vi "FTW-Linker-DecodeBitmap.vi"(7 "LinkerInfo":T7 {"iState" format="%08x"; "iStyle" format="%08x"; "wStyle" format="%08x"; "buttons" format="%08x"; "viflags" format="%08x"; "viflags2" format="%08x"}) -> (3 "iState":T6, 4 "viflags":T5, 6 "viflags2":T4, 8 "All Flags":bool[](array[boolean]), 10 "iStyle":T3, 14 "buttons":T1, 15 "wStyle":T2)   [LabVIEW 2015]
uses:
  FTW-Linker-LinkerInfoStructure.ctl
  FTW-Linker-LabVIEWFiletype.ctl
  FTW-Linker-Flags-iState.ctl
  FTW-Linker-Flags-viflags.ctl
  FTW-Linker-Flags-viflags2.ctl
  FTW-Linker-Flags-iStyle.ctl
  FTW-Linker-Flags-wStyle.ctl
  FTW-Linker-Flags-buttons.ctl
panel:
  # "Inputs"
  # "Outputs"
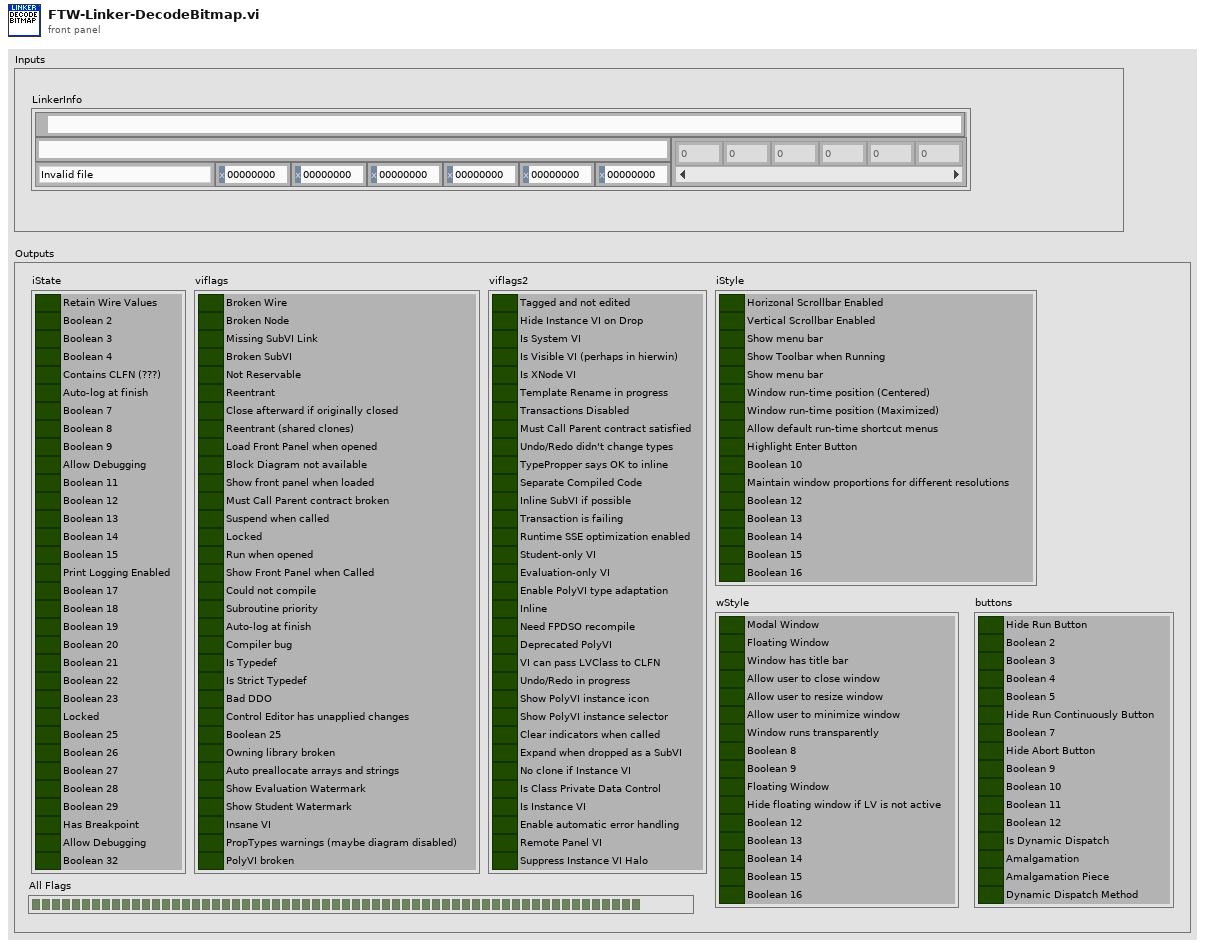
[diagram p1: front panel]
types:
  T1 = typedef "FTW-Linker-Flags-buttons.ctl" = cluster{"Hide Run Button":bool, "Boolean 2":bool, "Boolean 3":bool, "Boolean 4":bool, "Boolean 5":bool, "Hide Run Continuously Button":bool, "Boolean 7":bool, "Hide Abort Button":bool, "Boolean 9":bool, "Boolean 10":bool, "Boolean 11":bool, "Boolean 12":bool, "Is Dynamic Dispatch":bool, "Amalgamation":bool, "Amalgamation Piece":bool, "Dynamic Dispatch Method":bool}
  T2 = typedef "FTW-Linker-Flags-wStyle.ctl" = cluster{"Modal Window":bool, "Floating Window":bool, "Window has title bar":bool, "Allow user to close window":bool, "Allow user to resize window":bool, "Allow user to minimize window":bool, "Window runs transparently":bool, "Boolean 8":bool, "Boolean 9":bool, "Floating Window":bool, "Hide floating window if LV is not active":bool, "Boolean 12":bool, "Boolean 13":bool, "Boolean 14":bool, "Boolean 15":bool, "Boolean 16":bool}
  T3 = typedef "FTW-Linker-Flags-iStyle.ctl" = cluster{"Horizonal Scrollbar Enabled":bool, "Vertical Scrollbar Enabled":bool, "Show menu bar":bool, "Show Toolbar when Running":bool, "Show menu bar":bool, "Window run-time position (Centered)":bool, "Window run-time position (Maximized)":bool, "Allow default run-time shortcut menus":bool, "Highlight Enter Button":bool, "Boolean 10":bool, "Maintain window proportions for different resolutions":bool, "Boolean 12":bool, "Boolean 13":bool, "Boolean 14":bool, "Boolean 15":bool, "Boolean 16":bool}
  T4 = typedef "FTW-Linker-Flags-viflags2.ctl" = cluster{"Tagged and not edited":bool, "Hide Instance VI on Drop":bool, "Is System VI":bool, "Is Visible VI (perhaps in hierwin)":bool, "Is XNode VI":bool, "Template Rename in progress":bool, "Transactions Disabled":bool, "Must Call Parent contract satisfied":bool, "Undo/Redo didn't change types":bool, "TypePropper says OK to inline":bool, "Separate Compiled Code":bool, "Inline SubVI if possible":bool, "Transaction is failing":bool, "Runtime SSE optimization enabled":bool, "Student-only VI":bool, "Evaluation-only VI":bool, "Enable PolyVI type adaptation":bool, "Inline":bool, "Need FPDSO recompile":bool, "Deprecated PolyVI":bool, "VI can pass LVClass to CLFN":bool, "Undo/Redo in progress":bool, "Show PolyVI instance icon":bool, "Show PolyVI instance selector":bool, "Clear indicators when called":bool, "Expand when dropped as a SubVI":bool, "No clone if Instance VI":bool, "Is Class Private Data Control":bool, "Is Instance VI":bool, "Enable automatic error handling":bool, "Remote Panel VI":bool, "Suppress Instance VI Halo":bool}
  T5 = typedef "FTW-Linker-Flags-viflags.ctl" = cluster{"Broken Wire":bool, "Broken Node":bool, "Missing SubVI Link":bool, "Broken SubVI":bool, "Not Reservable":bool, "Reentrant":bool, "Close afterward if originally closed":bool, "Reentrant (shared clones)":bool, "Load Front Panel when opened":bool, "Block Diagram not available":bool, "Show front panel when loaded":bool, "Must Call Parent contract broken":bool, "Suspend when called":bool, "Locked":bool, "Run when opened":bool, "Show Front Panel when Called":bool, "Could not compile":bool, "Subroutine priority":bool, "Auto-log at finish":bool, "Compiler bug":bool, "Is Typedef":bool, "Is Strict Typedef":bool, "Bad DDO":bool, "Control Editor has unapplied changes":bool, "Boolean 25":bool, "Owning library broken":bool, "Auto preallocate arrays and strings":bool, "Show Evaluation Watermark":bool, "Show Student Watermark":bool, "Insane VI":bool, "PropTypes warnings (maybe diagram disabled)":bool, "PolyVI broken":bool}
  T6 = typedef "FTW-Linker-Flags-iState.ctl" = cluster{"Retain Wire Values":bool, "Boolean 2":bool, "Boolean 3":bool, "Boolean 4":bool, "Contains CLFN (???)":bool, "Auto-log at finish":bool, "Boolean 7":bool, "Boolean 8":bool, "Boolean 9":bool, "Allow Debugging":bool, "Boolean 11":bool, "Boolean 12":bool, "Boolean 13":bool, "Boolean 14":bool, "Boolean 15":bool, "Print Logging Enabled":bool, "Boolean 17":bool, "Boolean 18":bool, "Boolean 19":bool, "Boolean 20":bool, "Boolean 21":bool, "Boolean 22":bool, "Boolean 23":bool, "Locked":bool, "Boolean 25":bool, "Boolean 26":bool, "Boolean 27":bool, "Boolean 28":bool, "Boolean 29":bool, "Has Breakpoint":bool, "Allow Debugging":bool, "Boolean 32":bool}
  T7 = typedef "FTW-Linker-LinkerInfoStructure.ctl" = cluster{"path":path, "delimited name":string, "Filetype":T8, "iState":u32, "iStyle":u16, "wStyle":u16, "buttons":u16, "viflags":u32, "viflags2":u32, "links":u32[]}
  T8 = typedef "FTW-Linker-LabVIEWFiletype.ctl" = enum32{"Invalid file", "Unknown type", "VI", "Control", "PolyVI", "Project", "Library", "LVClass", "XControl", "XNode", "Shared Library", "dotNET assembly", "ActiveX interface", "CIN", "Run-time menu", "Palette menu", "Help file", "LLB", "XNode Edit Dependency", "LVClass Private Data", "Statechart", "MathScript .m file", "Ladder Diagram", "Packed Project Lib", "XNode Build Dependency"}
  T9 = cluster{"Boolean array[0]":bool, "Boolean array[1]":bool, "Boolean array[2]":bool, "Boolean array[3]":bool, "Boolean array[4]":bool, "Boolean array[5]":bool, "Boolean array[6]":bool, "Boolean array[7]":bool, "Boolean array[8]":bool, "Boolean array[9]":bool, "Boolean array[10]":bool, "Boolean array[11]":bool, "Boolean array[12]":bool, "Boolean array[13]":bool, "Boolean array[14]":bool, "Boolean array[15]":bool}
  T10 = cluster{"Boolean array[0]":bool, "Boolean array[1]":bool, "Boolean array[2]":bool, "Boolean array[3]":bool, "Boolean array[4]":bool, "Boolean array[5]":bool, "Boolean array[6]":bool, "Boolean array[7]":bool, "Boolean array[8]":bool, "Boolean array[9]":bool, "Boolean array[10]":bool, "Boolean array[11]":bool, "Boolean array[12]":bool, "Boolean array[13]":bool, "Boolean array[14]":bool, "Boolean array[15]":bool, "Boolean array[16]":bool, "Boolean array[17]":bool, "Boolean array[18]":bool, "Boolean array[19]":bool, "Boolean array[20]":bool, "Boolean array[21]":bool, "Boolean array[22]":bool, "Boolean array[23]":bool, "Boolean array[24]":bool, "Boolean array[25]":bool, "Boolean array[26]":bool, "Boolean array[27]":bool, "Boolean array[28]":bool, "Boolean array[29]":bool, "Boolean array[30]":bool, "Boolean array[31]":bool}
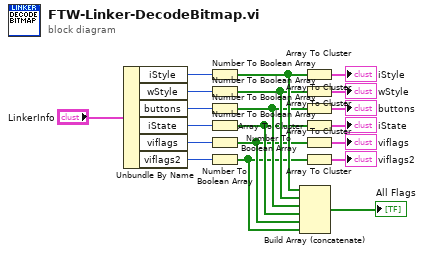
[diagram p0: block diagram]
diagram:
  n1 = Unbundle By Name("LinkerInfo") -> ("iStyle"=w6:u16, "wStyle"=w5:u16, "buttons"=w4:u16, "iState"=w3:u32, "viflags"=w2:u32, "viflags2"=w1:u32)
  n2 = Number To Boolean Array(number=w6) -> (Boolean array=w13:bool[])
  n3 = Number To Boolean Array(number=w5) -> (Boolean array=w12:bool[])
  n4 = Number To Boolean Array(number=w4) -> (Boolean array=w11:bool[])
  n5 = Number To Boolean Array(number=w3) -> (Boolean array=w10:bool[])
  n6 = Number To Boolean Array(number=w2) -> (Boolean array=w9:bool[])
  n7 = Number To Boolean Array(number=w1) -> (Boolean array=w8:bool[])
  n8 = Build Array (concatenate)(w13, w12, w11, w10, w9, w8) -> (→"All Flags":bool[])
  n9 = Array To Cluster(array=w13) -> (cluster=→"iStyle":T9)
  n10 = Array To Cluster(array=w12) -> (cluster=→"wStyle":T9)
  n11 = Array To Cluster(array=w11) -> (cluster=→"buttons":T9)
  n12 = Array To Cluster(array=w10) -> (cluster=→"iState":T10)
  n13 = Array To Cluster(array=w9) -> (cluster=→"viflags":T10)
  n14 = Array To Cluster(array=w8) -> (cluster=→"viflags2":T10)
